vi "Close_Popup.vi"(0 "Reference_In":refnum<vi>, 11 "Error_In":errorcluster) -> (4 "Reference_Out":refnum<vi>, 15 "Error_Out":errorcluster)   [LabVIEW 2023]
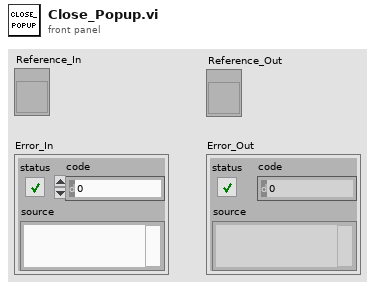
[diagram p1: front panel]
types:
  T1 = enum32{"Bad", "Idle", "Run top level", "Running"}
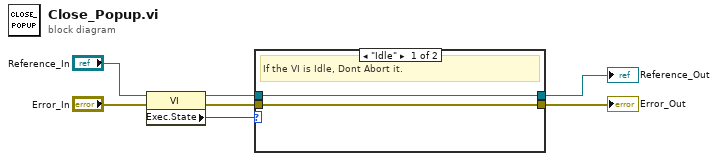
[diagram p0: block diagram]
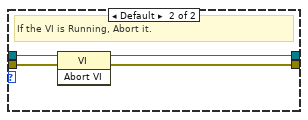
[diagram p2: hidden frame]
diagram:
  n1 = property on="Property Node" class="VI"(reference="Reference_In", error in="Error_In") -> (reference out=w7:refnum<vi>, error out=w6:errorcluster, "Exec.State"=w5:T1)
  n2 = case shown="\"Idle\"" w5 {
    tunnel: w7 -> [w9 w13]
    tunnel: w6 -> [w8 w12]
    tunnel: [w9 w11] -> w2
    tunnel: [w8 w10] -> w3
    frame "Idle" {
      # "If the VI is Idle, Dont Abort it."
    }
    frame Default {
      # "If the VI is Running, Abort it."
      n3 = invoke on="Invoke Node" class="VI" method="Abort VI"(reference=w13, error in=w12) -> (reference out=w11:refnum<vi>, error out=w10:errorcluster)  [unwired: 1 in, 1 out]
    }
  }
  "Reference_Out" <- w2
  "Error_Out" <- w3
